vi "SetupZSpan.vi"(8 "error in (no error)":errorcluster, 10 "Center Freq (Hz)":dbl=13250000000.0 format="%#.6g", 11 "SpecA_MXA.lvclass":refnum<class "SpecA_MXA.lvclass">) -> (0 "error out":errorcluster, 3 "SpecA_MXA.lvclass":refnum<class "SpecA_MXA.lvclass">)   [LabVIEW 2014, in "SpecA_MXA.lvclass"]
uses:
  SpecA_MXA.lvclass
  SpecA_MXA.lvclass/SpecA_MXA.ctl
  <instrlib>/Agilent MXA Series/Public/Configure/Configure Frequency (Center Span).vi
  <instrlib>/Agilent MXA Series/Agilent MXA Series.lvlib
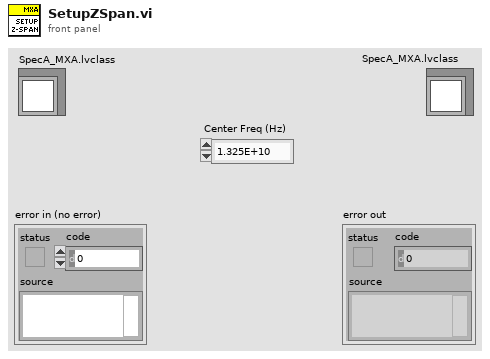
[diagram p1: front panel]
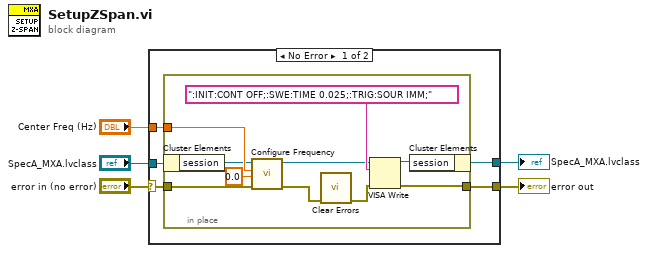
[diagram p0: block diagram]
diagram:
  n1 = case shown="No Error" "error in (no error)" {
    selector: "error in (no error)" -> [w6 w22]
    tunnel: "SpecA_MXA.lvclass" -> [w10 w21]
    tunnel: [w9 w21] -> w2
    tunnel: [w8 w22] -> w4
    tunnel: "Center Freq (Hz)" -> [w7 _]
    frame No Error {
      n2 = in-place {
        in-place-border: [w18] -> w8
        in-place-border: w7 -> [w19]
        in-place-border: w6 -> [w14]
        n3 = in-place-cluster #1(w10) -> ("session"=w15:refnum<visa-resource-name>)
        n4 = call-poly <instrlib>:"Configure Frequency.vi"("error in (no error)"=w14, "Span (2.65E+10 Hz)"=0.0, "Center Frequency (1.325E+10 Hz)"=w19, "VISA resource name"=w15) -> ("error out"=w12:errorcluster, "VISA resource name out"=w11:refnum<visa-resource-name>)  [unwired: 6 in]
        n5 = call <vilib>:"Clear Errors.vi"("error in (no error)"=w12) -> ("error out"=w13:errorcluster)  [unwired: 5 in, 1 out]
        n6 = VISA Write(VISA resource name=w11, write buffer=":INIT:CONT OFF;:SWE:TIME 0.025;:TRIG:SOUR IMM;" ("format string"), error in (no error)=w13) -> (VISA resource name out=w17:refnum<visa-resource-name>, error out=w18:errorcluster)  [unwired: 1 out]
        n7 = in-place-cluster #1("session"=w17) -> (w9:refnum<class "SpecA_MXA.lvclass">)
      }
    }
    frame Error {
    }
  }
  "error out" <- w4
  "SpecA_MXA.lvclass" <- w2
